vi "DISP err pack already finish.vi"(11 "result":string) -> (3 "étage3":bool)   [LabVIEW 2020]
uses:
  MsgBox.vi
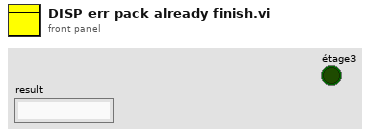
[diagram p1: front panel]
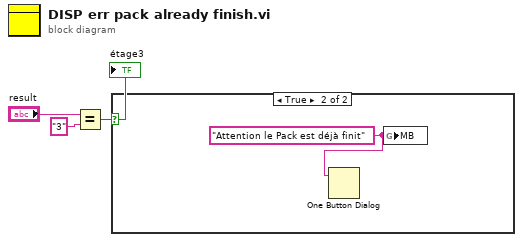
[diagram p0: block diagram]
diagram:
  n1 = Equal?(x="result", y="3") -> (x = y?=w3:bool)
  "étage3" <- w3
  n2 = case shown="True" w3 {
    frame False {
    }
    frame True {
      w4 = "Attention le Pack est déjà finit" ("MB")
      n3 = One Button Dialog(message=w4) -> ()  [unwired: 1 in, 1 out]
      n4 = global write "MsgBox.vi" "MB"(w4) -> ()
    }
  }
